vi "GetDescription.vi"(8 "Error In":errorcluster, 11 "reference in":refnum<class "TextDecorator.lvclass">) -> (0 "Error Out":errorcluster, 2 "Description":string, 3 "reference out":refnum<class "TextDecorator.lvclass">)   [LabVIEW 2024, in "TextDecorator.lvclass"]
uses:
  TextDecorator.lvclass
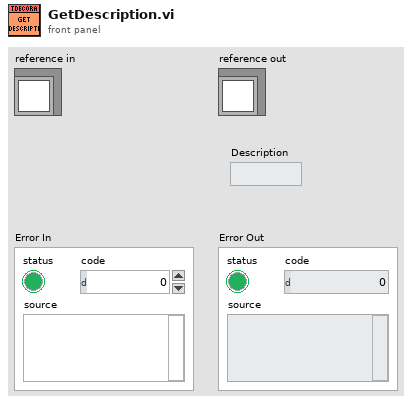
[diagram p1: front panel]
types:
  T1 = typedef "TextDecorator.lvclass/ObjectAttributes.ctl" = cluster{"TextRef":refnum<class "IText.lvclass">}
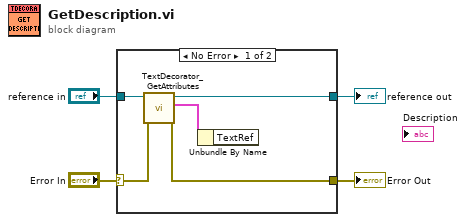
[diagram p0: block diagram]
diagram:
  n1 = case shown="No Error" "Error In" {
    selector: "Error In" -> [w9 w11]
    tunnel: [w7 w11] -> w3
    tunnel: [w5 w10] -> w1
    tunnel: "reference in" -> [w6 w10]
    frame No Error {
      n2 = call "TextDecorator_GetAttributes.vi"("Error In"=w9, "reference in"=w6) -> ("Error Out"=w7:errorcluster, "Data"=w8:T1, "reference out"=w5:refnum<class "TextDecorator.lvclass">)  [unwired: 6 in, 1 out]
      n3 = Unbundle By Name(w8) -> ()  [unwired: 1 out]
    }
    frame Error {
    }
  }
  "Error Out" <- w3
  "reference out" <- w1
